vi "Main.vi"() -> ()   [LabVIEW 2021]
doc: "This is the main VI that runs the pogram on MyRIO microcontroller. The user can choose the type of experiment to run, whether to attempt at stabilizing the ball at a desired coordinate or apply a PRBS signal to be later used to compute a frequency response model. The reference and actual paths as well as the controller input can be observed from th graphs on the front panel."
uses:
  system/System.lvclass
  <vilib>/Platform/TimedLoop/XDataNode/XDataNode.xnode
  <vilib>/Platform/TimedLoop/XDataNode/nitl_modes.ctl
  <vilib>/Platform/TimedLoop/XDataNode/XDNodeRunTimeDep.lvlib
  <vilib>/Platform/TimedLoop/XDataNode/wakeup.ctl
  <vilib>/Platform/TimedLoop/XDataNode/timing_clust.ctl
  system/mode.ctl
panel:
  in  "Option Tab":enum32{"Identify", "Control"}(tab)
  in  "PRBS":T1={"Frequency Divider"=5, "Periods"=8, "Order"=5, "Reference "=0, "Amplitude"=0.5} {"Amplitude" min=0.0; "Reference" items=["Change X", "Change Y"]; "Order" min=1 step=1; "Periods" min=1 step=1; "Frequency Divider" min=1 step=1}
  in  "Ref Point":cluster{"X Ref":dbl, "Y Ref":dbl} {"Y Ref" min=-8.0 max=8.0; "X Ref" min=-8.0 max=8.0}
  out "Y coordinate":cluster{"y":dbl, "y":dbl}(graph)
  out "X coordinate":cluster{"y":dbl, "y":dbl}(graph)
  in  "Controller Ref":path=path "/home/lvuser/Meebed/DDcontroller.bin"
  in  "Path logs":path=path "/home/lvuser/logs.bin"
  out "v":cluster{"y":dbl, "y":dbl}(graph)
  in  "Current Mode":T2
  out "error":errorcluster
  in  "stop":bool
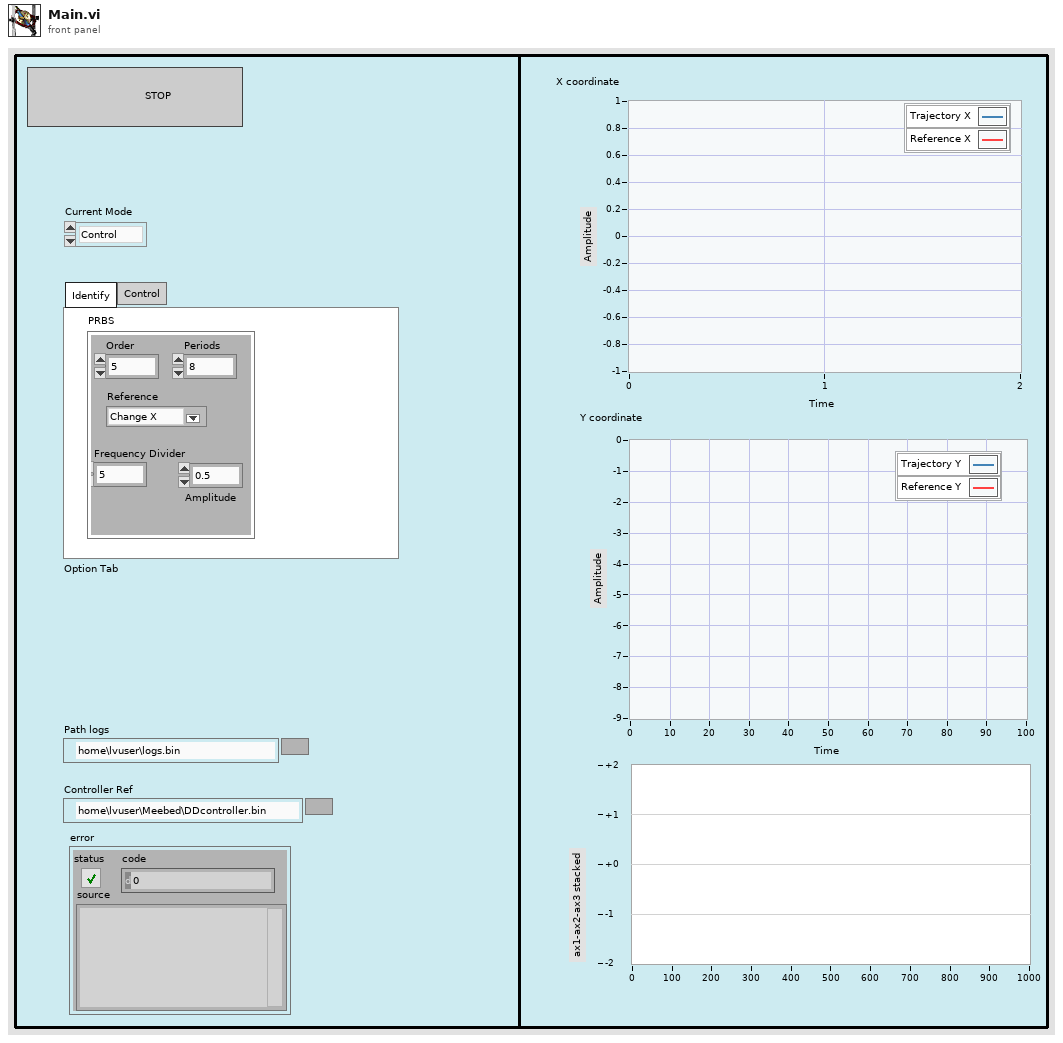
[diagram p1: front panel]
types:
  T1 = cluster{"Frequency Divider":u32, "Periods":u32, "Order":u32, "Reference ":u16, "Amplitude":dbl}
  T2 = typedef "System.lvclass/mode.ctl" = enum16{"Control", "Identify"}
  T3 = typedef "XDNodeRunTimeDep.lvlib/timing_clust.ctl" = cluster{"Expected End [f-1]":u64, "Actual End [f-1]":u64, "Finished Late? [f-1]":bool, "Expected End [i-1]":u64, "Actual End [i-1]":u64, "Finished Late? [i-1]":bool, "Expected Start [i]":u64, "Actual Start [i]":u64, "Expected Start [f]":u64, "Actual Start [f]":u64, "Source Name":string, "Structure Name":string, "Period":i64, "Deadline":i64, "Offset":i64, "Start":i64, "Priority":i32, "Timeout":i32, "Mode":T4, "Wakeup Reason":T5, "Error":errorcluster, "Source Type":string, "Secondary Source Type":string, "Global End Time":u64, "Global Start Time":u64, "Frame Duration":u64, "Iteration Duration":u64, "Assigned CPU":i32, "I/O Scan Engine Mode":u32}
  T4 = typedef "XDNodeRunTimeDep.lvlib/nitl_modes.ctl" = enum32{"No Change", "Process missed periods, maintain original phase", "Discard missed periods, maintain original phase", "Process missed periods, ignore original phase", "Discard missed periods, ignore original phase"}
  T5 = typedef "XDNodeRunTimeDep.lvlib/wakeup.ctl" = enum32{"Normal", "Aborted", "Asynchronous wakeup", "Timing source error", "Timed loop error", "Timeout"}
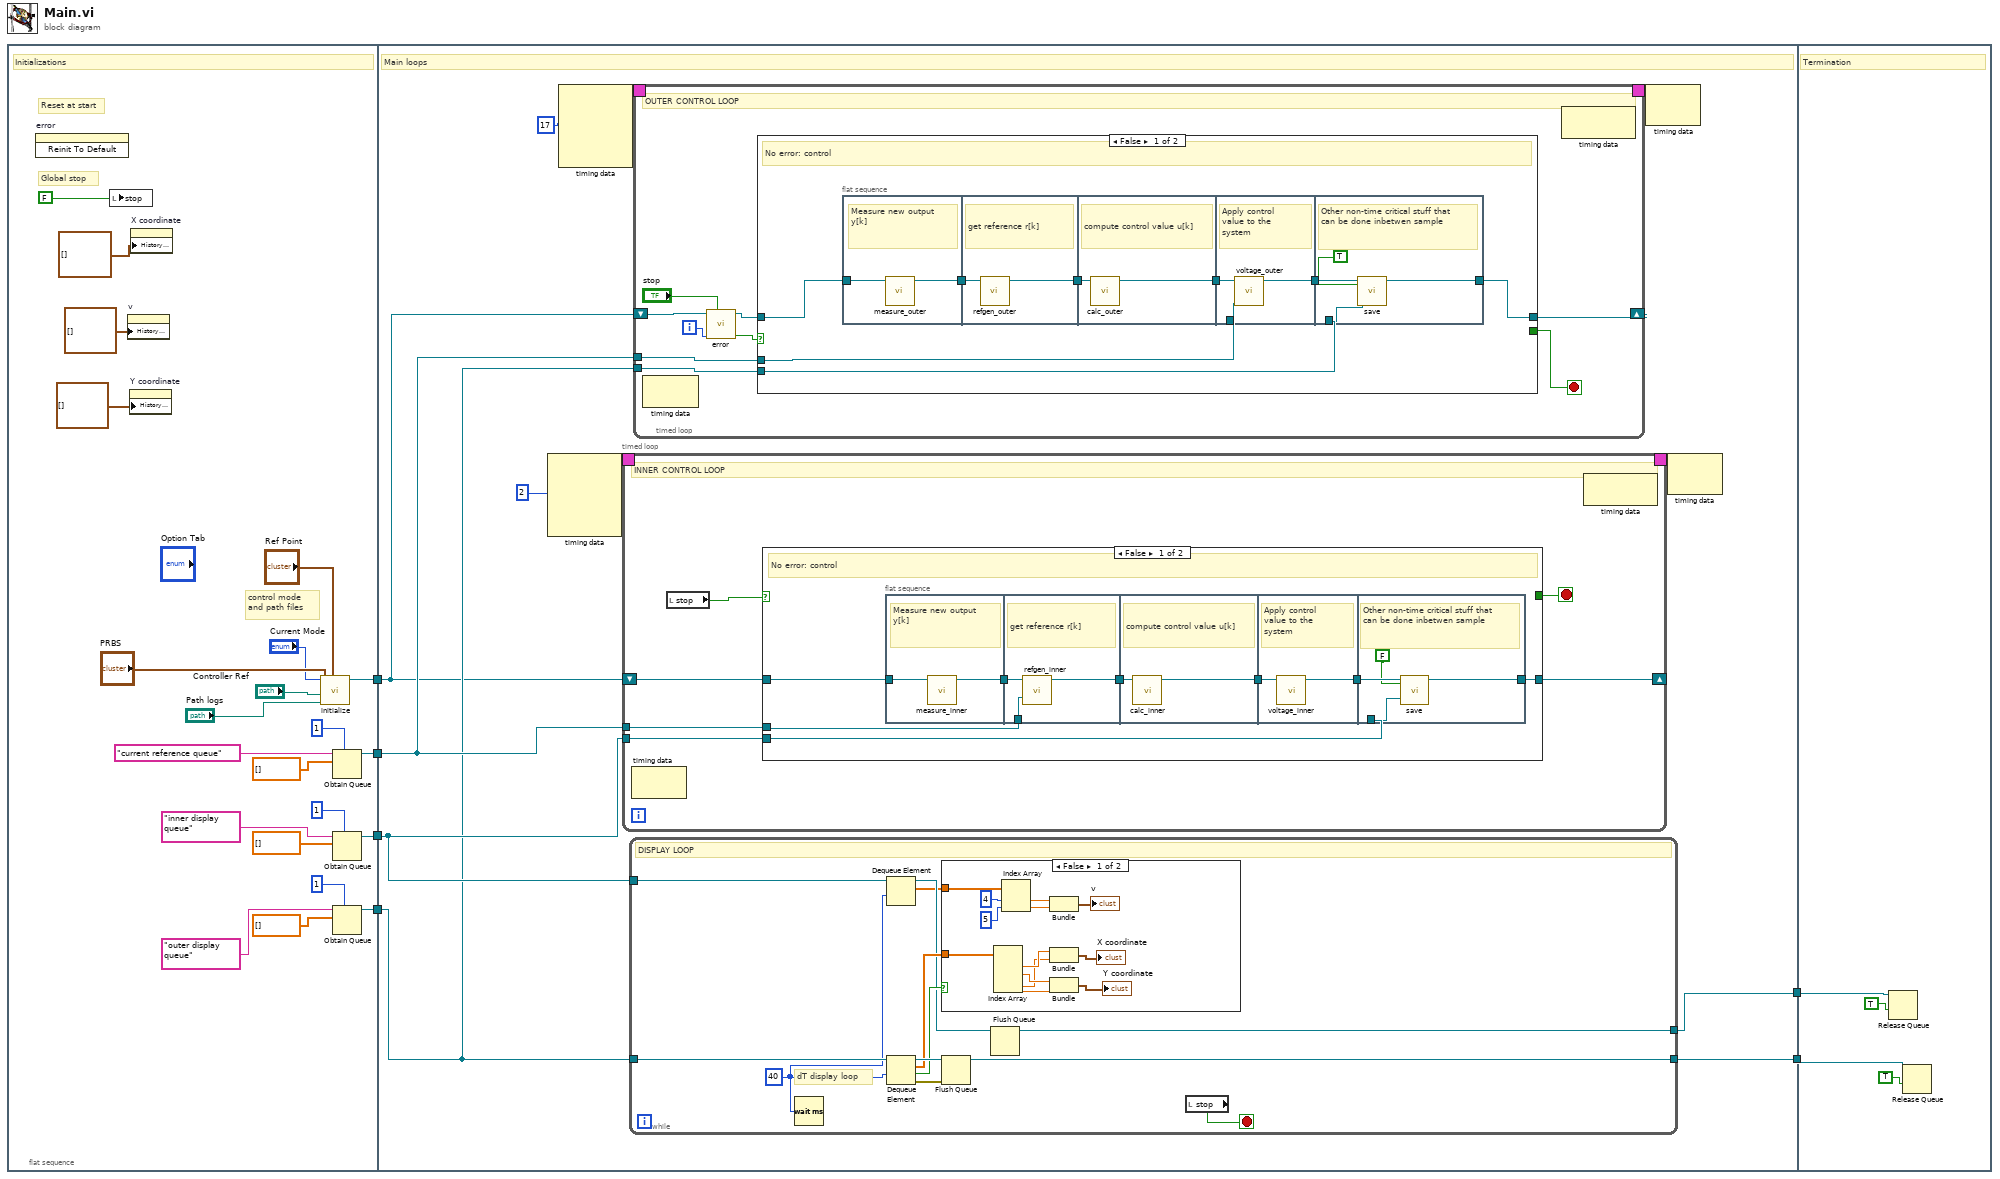
[diagram p0: block diagram]
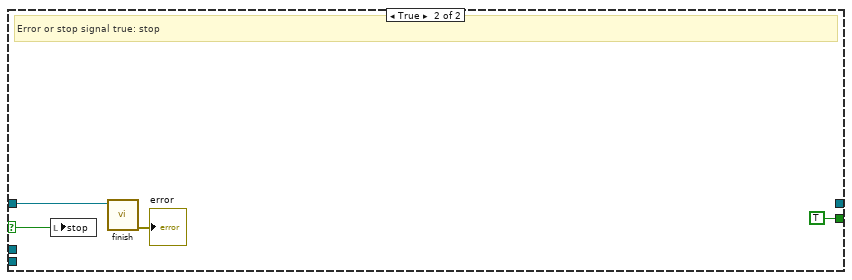
[diagram p3: hidden frame]
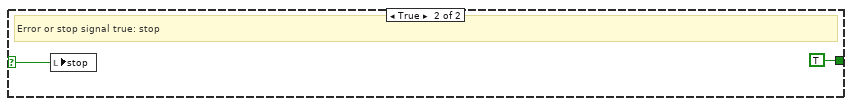
[diagram p4: hidden frame]
diagram:
  n1 = flat-sequence {
    tunnel: [w24] -> w6
    tunnel: [w28] -> w5
    tunnel: [w20] -> w4
    tunnel: [w14] -> w3
    tunnel: w6 -> [w30]
    tunnel: w5 -> [w31]
    tunnel: w4 -> [w32]
    tunnel: w3 -> [w37]
    tunnel: [w34] -> w2
    tunnel: [w29] -> w1
    tunnel: w2 -> [w142]
    tunnel: w1 -> [w141]
    frame #0 {
      # "control mode \nand path files"
      # "Reset at start"
      # "Global stop"
      # "Initializations"
      n2 = invoke on="error" class="Clust (strict)" method="Reinit To Default"() -> ()  [unwired: 3 in, 3 out]
      n3 = local write "stop"(FALSE ("stop")) -> ()
      n4 = property on="v" class="WFChart (strict)"("History Data"=cluster{"y":dbl, "y":dbl}[] []) -> ()  [unwired: 2 in, 2 out]
      n5 = property on="Y coordinate" class="WFChart (strict)"("History Data"=cluster{"y":dbl, "y":dbl}[] []) -> ()  [unwired: 2 in, 2 out]
      n6 = property on="X coordinate" class="WFChart (strict)"("History Data"=cluster{"y":dbl, "y":dbl}[] []) -> ()  [unwired: 2 in, 2 out]
      n7 = call "initialize.vi"("Ref Point"="Ref Point", "Data Savefile Path"="Path logs", "path refs"="Controller Ref", "Cluster"="PRBS", "mode"="Current Mode") -> ("Qube"=w24:refnum<class "System.lvclass">)  [unwired: 6 in]
      n8 = Obtain Queue(max queue size (-1, unlimited)=1, name (unnamed)="current reference queue", element data type=dbl[] [] ("y")) -> (queue out=w20:refnum<queue>)  [unwired: 2 in, 2 out]
      n9 = Obtain Queue(max queue size (-1, unlimited)=1, name (unnamed)="inner display queue", element data type=dbl[] [] ("y")) -> (queue out=w14:refnum<queue>)  [unwired: 2 in, 2 out]
      n10 = Obtain Queue(max queue size (-1, unlimited)=1, name (unnamed)="outer display queue", element data type=dbl[] [] ("y")) -> (queue out=w28:refnum<queue>)  [unwired: 2 in, 2 out]
    }
    frame #1 {
      # "Main loops"
      n11 = node-c288(i64 2 ("Period")) -> (w40:T3)  [unwired: 3 in]
      n12 = node-c288(i64 17 ("Period")) -> (w36:T3)  [unwired: 3 in]
      n13 = timed-loop {
        timing: w40 -> [_]
        timing-out: [_] -> w39
        shift-right: [w109] -> _
        shift-left: w30 -> [w111]
        tunnel: w37 -> [w108]
        tunnel: w32 -> [w107]
        stop <- w110 stop-if-true
        # "INNER CONTROL LOOP"
        n14 = node-c288() -> ()  [unwired: 1 in, 1 out]
        n15 = local read "stop"() -> (w106:bool)
        n16 = case shown="False" w106 {
          selector: w106 -> [_ w133]
          tunnel: w111 -> [w117 _]
          tunnel: [_ TRUE] -> w110
          tunnel: [w114 _] -> w109
          tunnel: w107 -> [w113 _]
          tunnel: w108 -> [w112 _]
          frame False {
            # "No error: control"
            n17 = flat-sequence {
              tunnel: [w120] -> w116
              tunnel: w117 -> [w121]
              tunnel: w116 -> [w124]
              tunnel: [w123] -> w115
              tunnel: w113 -> [w122]
              tunnel: [w125] -> w118
              tunnel: w115 -> [w126]
              tunnel: [w127] -> w119
              tunnel: w118 -> [w128]
              tunnel: w119 -> [w132]
              tunnel: [w130] -> w114
              tunnel: w112 -> [w129]
              frame #0 {
                # "Measure new output y[k]"
                n18 = call "measure_inner.vi"("Qube"=w121) -> ("Qube"=w120:refnum<class "System.lvclass">)  [unwired: 10 in]
              }
              frame #1 {
                # "get reference r[k]"
                n19 = call "refgen_inner.vi"("queue in"=w122, "Qube"=w124) -> ("Qube"=w123:refnum<class "System.lvclass">)  [unwired: 9 in]
              }
              frame #2 {
                # "compute control value u[k]"
                n20 = call "calc_inner.vi"("Qube"=w126) -> ("Qube"=w125:refnum<class "System.lvclass">)  [unwired: 10 in]
              }
              frame #3 {
                # "Apply control \nvalue to the system"
                n21 = call "voltage_inner.vi"("Qube"=w128) -> ("Qube"=w127:refnum<class "System.lvclass">)  [unwired: 10 in]
              }
              frame #4 {
                # "Other non-time critical stuff that can be done inbetwen sample"
                n22 = call "save.vi"("log?"=FALSE, "queue in"=w129, "Qube"=w132) -> ("Qube"=w130:refnum<class "System.lvclass">)  [unwired: 8 in]
              }
            }
          }
          frame True {
            # "Error or stop signal true: stop"
            n23 = local write "stop"(w133) -> ()
          }
        }
        n24 = node-c288() -> ()  [unwired: 1 in, 1 out]
      }
      n25 = while {
        tunnel: w31 -> [w51]
        tunnel: [w49] -> w34
        tunnel: w37 -> [w45]
        tunnel: [w42] -> w29
        stop <- w52 stop-if-true
        w44 = u32 40 ("Ts")
        # "dT display loop"
        # "DISPLAY LOOP"
        n26 = Wait (ms)(milliseconds to wait=w44) -> ()  [unwired: 1 out]
        n27 = Dequeue Element(queue=w45, timeout in ms (-1)=w44) -> (queue out=w43:refnum<queue>, element=w41:dbl[])  [unwired: 1 in, 2 out]
        n28 = Dequeue Element(queue=w51, timeout in ms (-1)=w44) -> (queue out=w50:refnum<queue>, element=w46:dbl[], timed out?=w47:bool, error out=w48:errorcluster)  [unwired: 1 in]
        n29 = case shown="False" w47 {
          tunnel: w46 -> [w65 _]
          tunnel: w41 -> [w63 _]
          frame False {
            n30 = Index Array(array=w65) -> (element #1=w64:dbl, element #2=w55:dbl, element #3=w54:dbl, element #4=w60:dbl)  [unwired: 4 in]
            n31 = Index Array(array=w63, index #1=4 ("index"), index #2=5 ("index")) -> (element #1=w59:dbl, element #2=w58:dbl)
            n32 = Bundle("y"=w59, "y"=w58) -> (→"v":cluster{"y":dbl, "y":dbl})  [unwired: 1 in]
            n33 = Bundle("y"=w64, "y"=w54) -> (→"X coordinate":cluster{"y":dbl, "y":dbl})  [unwired: 1 in]
            n34 = Bundle("y"=w55, "y"=w60) -> (→"Y coordinate":cluster{"y":dbl, "y":dbl})  [unwired: 1 in]
          }
          frame True {
          }
        }
        n35 = Flush Queue(queue=w50, error in (no error)=w48) -> (queue out=w49:refnum<queue>)  [unwired: 2 out]
        n36 = Flush Queue(queue=w43) -> (queue out=w42:refnum<queue>)  [unwired: 1 in, 2 out]
        n37 = local read "stop"() -> (w52:bool)
      }
      n38 = timed-loop {
        tunnel: w31 -> [w73]
        timing: w36 -> [_]
        timing-out: [_] -> w35
        shift-right: [w68] -> _
        shift-left: w30 -> [w71]
        tunnel: w32 -> [w67]
        i -> [w69]
        stop <- w74 stop-if-true
        # "OUTER CONTROL LOOP"
        n39 = node-c288() -> ()  [unwired: 1 in, 1 out]
        n40 = call "error.vi"("stop"="stop", "idx"=w69, "Qube"=w71) -> ("abort?"=w66:bool, "Qube"=w72:refnum<class "System.lvclass">)  [unwired: 7 in]
        n41 = case shown="False" w66 {
          selector: w66 -> [_ w99]
          tunnel: w72 -> [w82 w100]
          tunnel: [_ TRUE] -> w74
          tunnel: w73 -> [w79 _]
          tunnel: [w78 _] -> w68
          tunnel: w67 -> [w77 _]
          frame False {
            # "No error: control"
            n42 = flat-sequence {
              tunnel: [w85] -> w81
              tunnel: w82 -> [w86]
              tunnel: w81 -> [w87]
              tunnel: [w88] -> w80
              tunnel: [w90] -> w83
              tunnel: w80 -> [w89]
              tunnel: [w93] -> w84
              tunnel: w83 -> [w92]
              tunnel: w77 -> [w91]
              tunnel: w84 -> [w97]
              tunnel: w79 -> [w94]
              tunnel: [w95] -> w78
              frame #0 {
                # "Measure new output y[k]"
                n43 = call "measure_outer.vi"("Qube"=w86) -> ("Qube"=w85:refnum<class "System.lvclass">)  [unwired: 10 in]
              }
              frame #1 {
                # "get reference r[k]"
                n44 = call "refgen_outer.vi"("Qube"=w87) -> ("Qube"=w88:refnum<class "System.lvclass">)  [unwired: 10 in]
              }
              frame #2 {
                # "compute control value u[k]"
                n45 = call "calc_outer.vi"("Qube"=w89) -> ("Qube"=w90:refnum<class "System.lvclass">)  [unwired: 10 in]
              }
              frame #3 {
                # "Apply control \nvalue to the system"
                n46 = call "voltage_outer.vi"("queue"=w91, "Qube"=w92) -> ("Qube"=w93:refnum<class "System.lvclass">)  [unwired: 9 in]
              }
              frame #4 {
                # "Other non-time critical stuff that can be done inbetwen sample"
                n47 = call "save.vi"("log?"=TRUE, "queue in"=w94, "Qube"=w97) -> ("Qube"=w95:refnum<class "System.lvclass">)  [unwired: 8 in]
              }
            }
          }
          frame True {
            # "Error or stop signal true: stop"
            n48 = local write "stop"(w99) -> ()
            n49 = call "finish.vi"("ActiveSuspension.lvclass"=w100) -> ("error out"=→"error":errorcluster)  [unwired: 10 in]
          }
        }
        n50 = node-c288() -> ()  [unwired: 1 in, 1 out]
      }
      n51 = node-c288(w35) -> ()  [unwired: 1 out]
      n52 = node-c288(w39) -> ()  [unwired: 1 out]
    }
    frame #2 {
      # "Termination"
      n53 = Release Queue(queue=w141, force destroy? (F)=TRUE) -> ()  [unwired: 1 in, 3 out]
      n54 = Release Queue(queue=w142, force destroy? (F)=TRUE) -> ()  [unwired: 1 in, 3 out]
    }
  }
